vi "L0_SUMnADDS_NOISE_TEST.vi"() -> ()   [LabVIEW 2012]
uses:
  <vilib>/Utility/NIReport.llb/NI_report.lvclass
  <vilib>/Utility/NIReport.llb/HTML/NI_HTML.lvclass
  <instrlib>/Agilent 8000 Series/Public/Configure/Configure Math (Binary Operation).vi
  L0&L1/L0_BOARD_TESTs/trunk/Sum_Abrilader/L0_Sum_Adder Folder/C/Program Files/National Instruments/LabVIEW 2012/instr.lib/Agilent 8000 Series/Public/Data/Low Level/Fetch Measurement (More).vi
  <instrlib>/Agilent 8000 Series/Agilent 8000 Series.lvlib
panel:
  in  "Serial Number":string="SN_026"
  in  "SET 2?":bool
  in  "SET?":bool=TRUE
  in  "Clip_sel_b":u32=1
  in  "Ib_ClipVb":u32=63
  in  "Att gain":u32
  in  "Delay Enable":i32
  in  "Gen Active":bool
  in  "Control\nGenNOsc":bool=TRUE
  in  "Amp Scaler":dbl(slide)=112.5152621432011 scale=0.1..250.0
  in  "Voltage Input":dbl(slide)=0.33316326530612245 scale=0.05..0.8
  in  "Channels \nCombinations":i32[](array[numeric])=[3, 12, 48, 96, 7, 28, 112, 15, 120, 31, 124, 63, 126, 127]
  out "element":i32=127
  in  "Instrument VISA in":T1={"AWG VISA"="AgilentGenerator1", "Oscilloscope  VISA "="AgilentOsciloscope", "Integration Board IP"="172.16.17.47", "connection ID"=refnum, "report out"=refnum, "report file path"=path "C:/Users/omartinez/Desktop/L0nL1_Results"}
  out "error out":errorcluster={"status"=FALSE, "code"=-1074000000, "source"="Agilent 8000 Series.lvlib:Error Query.vi<ERR>\nInstrument reports:\n-222,\"Data out of range\"\r\n0,\"No error\"\r\n\n\n\n<b>Complete call chain:</b>\r\n     Agilent 8000 Series.lvlib:Error Query.vi\r\n     Agilent 8000 Series.lvlib:Configure Channel.vi\r\n     SetGenNOscNoise.vi\r\n     L0_SUMnADDS_NOISE_TEST.vi"}
  in  "error in (no error)":errorcluster
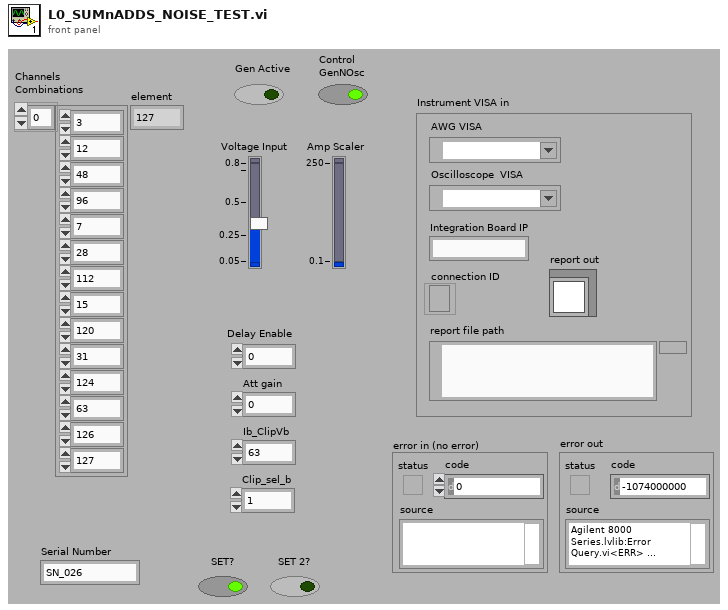
[diagram p1: front panel]
types:
  T1 = cluster{"AWG VISA":refnum<visa-resource-name>, "Oscilloscope  VISA ":refnum<visa-resource-name>, "Integration Board IP":string, "connection ID":refnum<k5>, "report out":refnum<class "NI_report.lvclass">, "report file path":path}
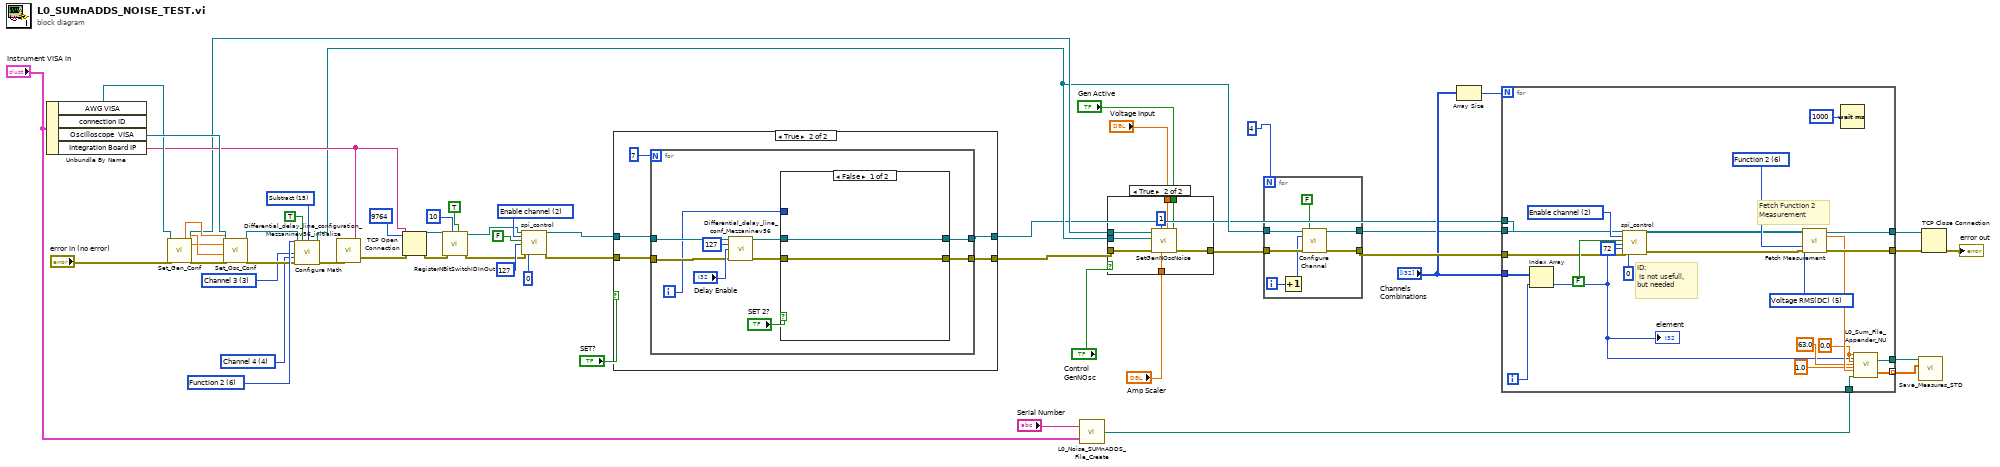
[diagram p0: block diagram]
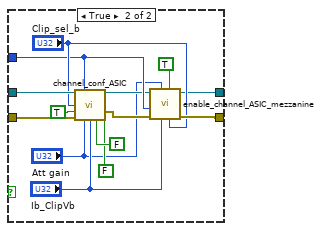
[diagram p4: hidden frame]
diagram:
  w25 = u16 2 items=["Attenuation", "Clipping", "Enable channel", "Delay line", "ASIC"] ("Device")
  w36 = u16 6 items=["Function 1"=5, "Function 2"=6, "Function 3"=7, "Function 4"=8] ("Math Channel (5: Function 1)")
  w37 = u16 15 items=["Add"=12, "Divide"=13, "Multiply"=14, "Subtract"=15, "Common Mode"=16, "Versus"=17] ("Math Operation (12: Add)")
  w31 = 3 items=["Channel 1"=1, "Channel 2"=2, "Channel 3"=3, "Channel 4"=4] ("Channel (1: Channel 1)")
  w32 = 4 items=["Channel 1"=1, "Channel 2"=2, "Channel 3"=3, "Channel 4"=4] ("Channel (1: Channel 1)")
  n1 = Unbundle By Name("Instrument VISA in") -> ("AWG VISA"=w49:refnum<visa-resource-name>, "Oscilloscope  VISA"=w50:refnum<visa-resource-name>, "Integration Board IP"=w39:string)  [unwired: 1 out]
  n2 = call "Set_Gen_Conf.vi"("AWG VISA"=w49, "error in (no error)"="error in (no error)") -> ("Amplitude 1 OUT"=w47:dbl, "VISA resource name out"=w28:refnum<visa-resource-name>, "Pulse Width in seconds 1 OUT"=w46:dbl, "Trigger Level 1"=w45:dbl, "error out"=w51:errorcluster)  [unwired: 10 in, 3 out]
  n3 = call "Set_Osc_Conf.vi"("VISA resource name"=w50, "Amplitude IN"=w47, "Trigger Level IN"=w45, "Pulse Width in seconds IN"=w46, "error in (no error)"=w51) -> ("VISA resource name out"=w35:refnum<visa-resource-name>, "error out"=w34:errorcluster)  [unwired: 13 in]
  n4 = call-poly <instrlib>:"Configure Math.vi"("VISA resource name"=w35, "Enable Math Channel (T:Enable)"=TRUE, "Math Operation (12: Add)"=w37, "Math Channel (5: Function 1)"=w36, "Math Operand (1: Channel 1)"=w31, "Math Operand (2: Channel 2)"=w32, "error in (no error)"=w34) -> ("VISA resource name out"=w10:refnum<visa-resource-name>, "error out"=w33:errorcluster)  [unwired: 7 in]
  n5 = call "Differential_delay_line_configuration_Mezzaninev56_initialize.vi"("error in (no error)"=w33, "address"=w39) -> ("error out 2"=w44:errorcluster)
  n6 = TCP Open Connection(address=w39, remote port or service name=9764, error in (no error)=w44) -> (connection ID=w42:refnum<k5>, error out=w43:errorcluster)  [unwired: 2 in]
  n7 = call "RegisterNBitSwitchIDInOut.vi"("Switch Bit"=TRUE, "N Bit"=10, "error in (no error)"=w43, "connection ID"=w42) -> ("error out"=w22:errorcluster, "connection ID out"=w19:refnum<k5>)  [unwired: 5 in]
  n8 = call "spi_control.vi"("connection ID"=w19, "Device"=w25, "Read/#write"=FALSE, "Data"=127, "error out 3"=w22, "Id in"=0) -> ("connection ID out"=w20:refnum<k5>, "error out 2"=w21:errorcluster)  [unwired: 6 in, 6 out]
  n9 = case shown="True" "SET?" {
    tunnel: [w55 w59] -> w27
    tunnel: [w54 w58] -> w1
    tunnel: w21 -> [w55 w57]
    tunnel: w20 -> [w54 w56]
    frame False {
    }
    frame True {
      n10 = for {
        N: 7 -> [_]
        tunnel: w57 -> [w69]
        tunnel: w56 -> [w68]
        tunnel: [w65] -> w59
        tunnel: [w63] -> w58
        i -> [w64]
        n11 = call "Differential_delay_line_conf_Mezzaninev56.vi"("connection ID"=w68, "channel"=127, "Delay value"="Delay Enable", "error in (no error)"=w69) -> ("connection ID out"=w66:refnum<k5>, "error out 2"=w67:errorcluster)  [unwired: 4 in, 6 out]
        n12 = case shown="False" "SET 2?" {
          tunnel: w67 -> [w72 w86]
          tunnel: w66 -> [w71 w85]
          tunnel: [w72 w80] -> w65
          tunnel: w64 -> [_ w77]
          tunnel: [w71 w73] -> w63
          frame False {
          }
          frame True {
            n13 = call "channel_conf_ASIC.vi"("connection ID"=w85, "Ring"=w77, "Clip_sel_b"="Clip_sel_b", "CompBuf_en_b"=TRUE, "error out"=w86, "Att gain"="Att gain", "Ib_ClipVb"="Ib_ClipVb", "Clip_en_b"=FALSE, "Att_en_b"=FALSE) -> ("connection ID out"=w76:refnum<k5>, "error out 2"=w81:errorcluster)  [unwired: 2 in, 3 out]
            n14 = call "enable_channel_ASIC_mezzanine.vi"("Clip_sel_b"="Clip_sel_b", "maj/sum"=TRUE, "Ib_clipVb"="Ib_ClipVb", "Att gain"="Att gain", "error in"=w81, "Channel"=w77, "connection ID"=w76) -> ("error out"=w80:errorcluster, "connection ID out"=w73:refnum<k5>)  [unwired: 2 in, 1 out]
          }
        }
      }
    }
  }
  n15 = call "L0_Noise_SUMnADDS_File_Create.vi"("input cluster"="Instrument VISA in", "Serial Number"="Serial Number") -> ("appended path"=w2:path)
  n16 = case shown="True" "Control\nGenNOsc" {
    tunnel: w10 -> [_ w95]
    tunnel: w28 -> [_ w94]
    tunnel: w27 -> [w87 w93]
    tunnel: [w87 w92] -> w12
    tunnel: "Voltage Input" -> [_ w90]
    tunnel: "Amp Scaler" -> [_ w89]
    tunnel: "Gen Active" -> [_ w88]
    frame False {
    }
    frame True {
      n17 = call "SetGenNOscNoise.vi"("Enable Output"=w88, "Input Voltage"=w90, "Amp Scaler"=w89, "NChannels"=1, "error in (no error)"=w93, "VISA resource name"=w95, "AWG VISA"=w94) -> ("error out 2"=w92:errorcluster)  [unwired: 4 in]
    }
  }
  n18 = for {
    N: 4 -> [_]
    tunnel: w12 -> [w102]
    tunnel: [w101] -> w11
    tunnel: w10 -> [w99]
    tunnel: [w96] -> w7
    i -> [w100]
    n19 = Increment(x=w100) -> (x+1=w97:i32)
    n20 = call <instrlib>:"Configure Channel.vi"("VISA resource name"=w99, "Enable Channel (Enable)"=FALSE, "Channel (1: Channel 1)"=w97, "error in (no error)"=w102) -> ("VISA resource name out"=w96:refnum<visa-resource-name>, "error out"=w101:errorcluster)  [unwired: 10 in]
  }
  n21 = Array Size(array="Channels \nCombinations") -> (size(s)=w9:i32)
  n22 = for {
    N: w9 -> [_]
    tunnel: [w115] -> w30
    tunnel: [w116] -> w29
    tunnel: "Channels \nCombinations" -> [w122]
    tunnel: w11 -> [w121]
    tunnel: w7 -> [w114]
    tunnel: [w109] -> w6 mode=indexing
    tunnel: [w108] -> w5
    tunnel: w2 -> [w107]
    tunnel: w1 -> [w103]
    i -> [w120]
    w112 = 0.0 ("Vin")
    w118 = 5 items=["Rise Time", "Fall Time", "Frequency", "Period", "Voltage RMS(AC)", "Voltage RMS(DC)", "Voltage RMS (AC,cycle)", "Voltage RMS (DC,cycle)", "Voltage Max", "Voltage Min", "Voltage Middle", "Voltage Vpp", "Voltage High", "Voltage Low", "Voltage Average", "Voltage Average (cycle)", "Width Negative", "Width Positive", "Duty Cycle Positive", "Amplitude", "Overshoot", "Preshoot", "Voltage Base", "Voltage Upper", "Time Max", "Time Min", "Color Grade Crossing", "Color Grade Eye Width", "Color Grade Eye Height", "Color Grade Eye Q-Factory", "Color Grade Eye Duty Cycle Distortion(Percent)", "Color Grade Eye Duty Cycle Distortion(Time)", "Color Grade Eye Jitter(PP)", "Color Grade Eye Width(RMS)", "Cycle-cycle Duty Jitter(Rising)", "Cycle-cycle Duty Jitter(Falling)", "Cycle-cycle Jitter(Rising)", "Cycle-cycle Jitter(Falling)", "Cycle-cycle - Width", "Cycle-cycle + Width", "Date Rate", "Unit Interval", "FFT Delta Frequency", "FFT Delta Magnitude", "FFT Frequency", "FFT Magnitude", "Slew Rate", "Area (Entire Display)", "Area(Single Cycle)", "Duty Cycle (Rising)", "Duty Cycle (Falling)"] ("Measurement Function (0: Rise Time)")
    w119 = 6 items=["Channel 1"=1, "Channel 2"=2, "Channel 3"=3, "Channel 4"=4, "Function 1"=5, "Function 2"=6, "Function 3"=7, "Function 4"=8, "Memory 1"=9, "Memory 2"=10, "Memory 3"=11, "Memory 4"=12] ("Channel (1: Channel 1)")
    w124 = u16 2 items=["Attenuation", "Clipping", "Enable channel", "Delay line", "ASIC"] ("Device")
    # "Fetch Function 2\nMeasurement"
    # "ID:\n Is not usefull, \nbut needed"
    n23 = Index Array(array=w122, index=w120) -> (element=w105:i32)
    "element" <- w105
    n24 = call "spi_control.vi"("connection ID"=w103, "Device"=w124, "Read/#write"=FALSE, "Data"=w105, "Register or channel"=72, "error out 3"=w121, "Id in"=0) -> ("connection ID out"=w115:refnum<k5>, "error out 2"=w117:errorcluster)  [unwired: 5 in, 6 out]
    n25 = call-poly "Fetch Measurement.vi"("VISA resource name"=w114, "Channel (1: Channel 1)"=w119, "Measurement Function (0: Rise Time)"=w118, "error in (no error)"=w117) -> ("Measurement"=w113:dbl, "error out"=w116:errorcluster)  [unwired: 9 in, 1 out]
    n26 = Wait (ms)(milliseconds to wait=u32 1000) -> ()  [unwired: 1 out]
    n27 = call "L0_Sum_File_Appender_NU.vi"("Vin"=w112, "CH"=w105, "Att"=w112, "IbClip"=63.0, "Clip"=1.0, "Vmeas"=w113, "file path (dialog if empty)"=w107) -> ("appended array"=w109:dbl[], "file path (dialog if empty) 2"=w108:path)  [unwired: 19 in]
  }
  n28 = call "Save_Measures_STD.vi"("Data in"=w6, "file path (dialog if empty)"=w5) -> ()  [unwired: 10 in]
  n29 = TCP Close Connection(connection ID=w30, error in (no error)=w29) -> (error out=→"error out":errorcluster)  [unwired: 1 in, 1 out]
